vi "convertLatLong.vi"(2 "Longitude (deg)":string, 3 "Latitude (deg)":string) -> (0 "Longitude (deg)":dbl, 1 "Latitude (deg)":dbl)   [LabVIEW 2015]
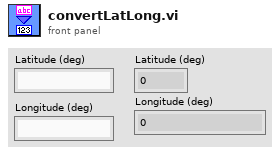
[diagram p1: front panel]
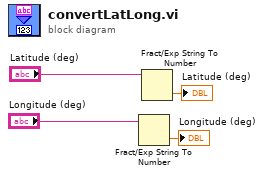
[diagram p0: block diagram]
diagram:
  n1 = Fract/Exp String To Number(string="Longitude (deg)") -> (number=→"Longitude (deg)":dbl)  [unwired: 3 in, 1 out]
  n2 = Fract/Exp String To Number(string="Latitude (deg)") -> (number=→"Latitude (deg)":dbl)  [unwired: 3 in, 1 out]
